vi "input-validation_v4.vi"(8 "error constant":errorcluster, 9 "Ki-xy":sgl=0.005, 11 "z_axis_params":T1={"z_u_max"=5.0, "setpoint-scan"=0.0, "Ki-scan"=0.001, "uz_safe"=0.0, "Kiz_down"=0.001, "setpoint-up"=0.0, "TF-params"={"TF-order"=0, "Num"=[0.0, 0.0, 0.0, 0.0, 0.0, 0.0, 0.0, 0.0, 0.0], "Den"=[0.0, 0.0, 0.0, 0.0, 0.0, 0.0, 0.0, 0.0, 0.0]}, "do-Dz"=FALSE, "PID-while-xy-move"=FALSE} {"Kiz_down" format="%#_13g"; "z_u_max" format="%#_13g"}) -> (0 "error out":errorcluster)   [LabVIEW 2017]
uses:
  controls/z-axis-params_v4_prescan.ctl
  controls/TF-params.ctl
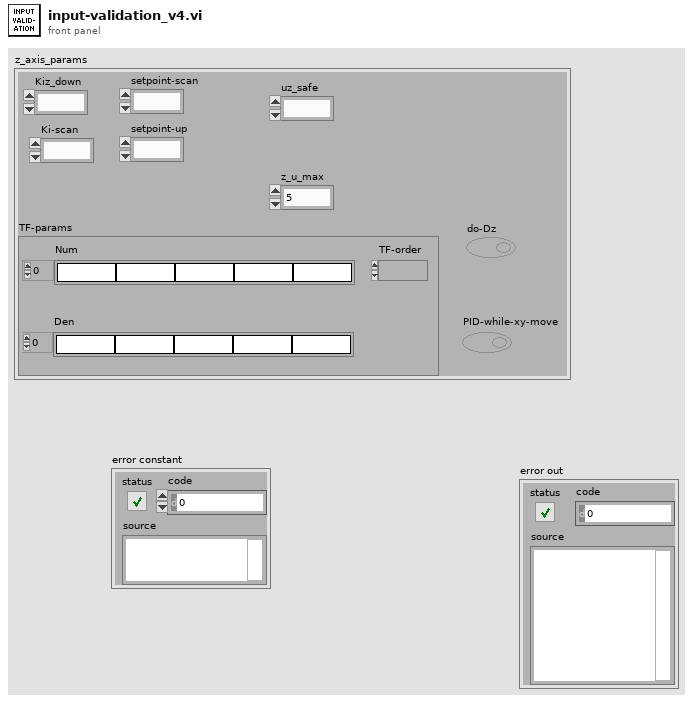
[diagram p1: front panel]
types:
  T1 = typedef "z-axis-params_v4_prescan.ctl" = cluster{"z_u_max":sgl, "setpoint-scan":fxp<+/-,32,16>, "Ki-scan":sgl, "uz_safe":fxp<+/-,16,5>, "Kiz_down":sgl, "setpoint-up":fxp<+/-,32,16>, "TF-params":T2, "do-Dz":bool, "PID-while-xy-move":bool}
  T2 = typedef "TF-params.ctl" = cluster{"TF-order":i16, "Num":sgl[], "Den":sgl[]}
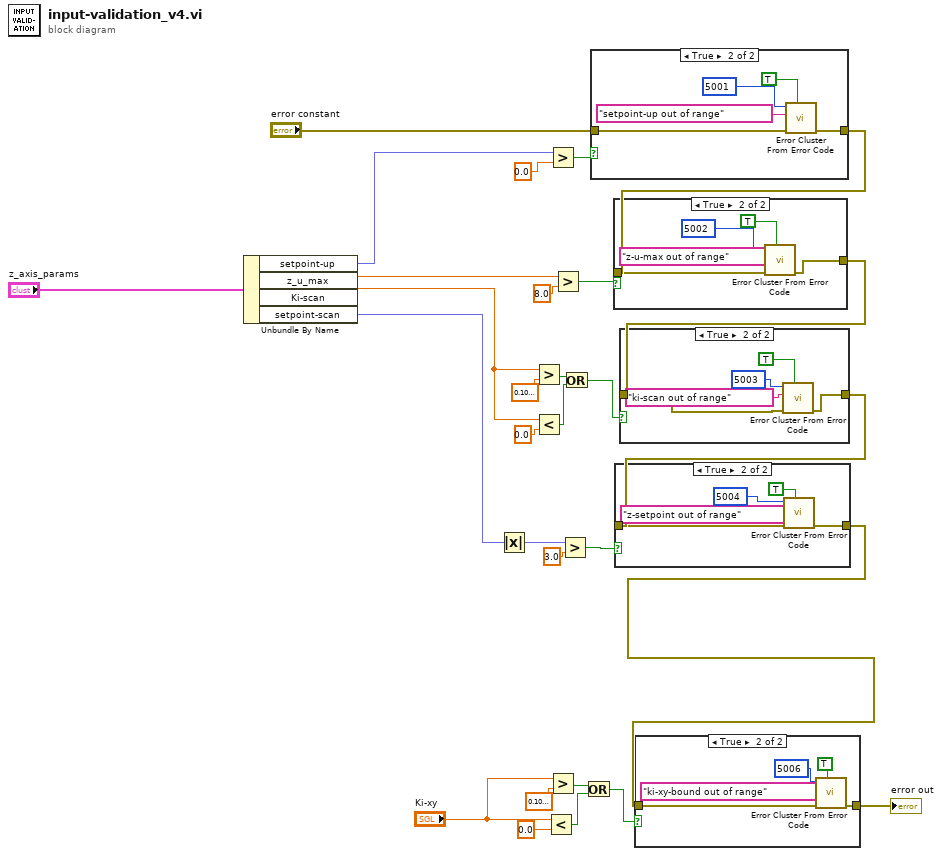
[diagram p0: block diagram]
diagram:
  n1 = Unbundle By Name("z_axis_params") -> ("setpoint-up"=w24:fxp<+/-,32,16>, "z_u_max"=w22:sgl, "Ki-scan"=w5:sgl, "setpoint-scan"=w4:fxp<+/-,32,16>)
  n2 = Absolute Value(x=w4) -> (abs(x)=w28:fxp<+,32,16>)
  n3 = Greater?(x=w5, y=sgl 0.1) -> (0:w13:bool)
  n4 = Less?(x=w5, y=sgl 0.0) -> (x < y?=w14:bool)
  n5 = Less?(x="Ki-xy", y=sgl 0.0) -> (x < y?=w8:bool)
  n6 = Greater?(x=w24, y=sgl 0.0) -> (0:w19:bool)
  n7 = Greater?(x="Ki-xy", y=sgl 0.1) -> (0:w9:bool)
  n8 = Greater?(x=w22, y=sgl 8.0) -> (0:w11:bool)
  n9 = Greater?(x=w28, y=sgl 3.0) -> (0:w15:bool)
  n10 = Or(x=w13, y=w14) -> (x .or. y?=w12:bool)
  n11 = Or(x=w9, y=w8) -> (x .or. y?=w7:bool)
  n12 = case shown="True" w19 {
    tunnel: "error constant" -> [w30 w35]
    tunnel: [w30 w31] -> w18
    frame False {
    }
    frame True {
      n13 = call <vilib>:"Error Cluster From Error Code.vi"("show call chain? (False)"=TRUE, "error in (no error)"=w35, "error message (\"\")"="setpoint-up out of range", "error code (0)"=5001) -> ("error out"=w31:errorcluster)  [unwired: 5 in]
    }
  }
  n14 = case shown="True" w11 {
    tunnel: w18 -> [w36 w39]
    tunnel: [w36 w40] -> w17
    frame False {
    }
    frame True {
      n15 = call <vilib>:"Error Cluster From Error Code.vi"("show call chain? (False)"=TRUE, "error in (no error)"=w39, "error message (\"\")"="z-u-max out of range", "error code (0)"=5002) -> ("error out"=w40:errorcluster)  [unwired: 5 in]
    }
  }
  n16 = case shown="True" w12 {
    tunnel: w17 -> [w42 w43]
    tunnel: [w42 w44] -> w16
    frame False {
    }
    frame True {
      n17 = call <vilib>:"Error Cluster From Error Code.vi"("show call chain? (False)"=TRUE, "error in (no error)"=w43, "error message (\"\")"="ki-scan out of range", "error code (0)"=5003) -> ("error out"=w44:errorcluster)  [unwired: 5 in]
    }
  }
  n18 = case shown="True" w15 {
    tunnel: w16 -> [w48 w51]
    tunnel: [w48 w52] -> w2
    frame False {
    }
    frame True {
      n19 = call <vilib>:"Error Cluster From Error Code.vi"("show call chain? (False)"=TRUE, "error in (no error)"=w51, "error message (\"\")"="z-setpoint out of range", "error code (0)"=5004) -> ("error out"=w52:errorcluster)  [unwired: 5 in]
    }
  }
  n20 = case shown="True" w7 {
    tunnel: [w54 w56] -> w3
    tunnel: w2 -> [w54 w57]
    frame False {
    }
    frame True {
      n21 = call <vilib>:"Error Cluster From Error Code.vi"("show call chain? (False)"=TRUE, "error in (no error)"=w57, "error message (\"\")"="ki-xy-bound out of range", "error code (0)"=5006) -> ("error out"=w56:errorcluster)  [unwired: 5 in]
    }
  }
  "error out" <- w3
